vi "M81 Read Values_Suslov.vi"(9 "Slot":enum32{"Slot 1", "Slot 2", "Slot 3"}(ring), 10 "Command string":string, 11 "VISA resource name":refnum<visa-resource-name>) -> (2 "Resistance":dbl[](array[numeric]), 3 "VISA resource name":refnum<visa-resource-name>)   [LabVIEW 2025]
doc: "Author: Scott Hannahs <sth@magnet.fsu.edu>\n\nThis software is licensed for use under the “MIT License\"\nCopyright (c) 2025 Scott Hannahs, sth@sth@magnet.sthnet.net\n\nPermission is hereby granted, free of charge, to any person obtaining a copy of this software and associated documentation files (the \"Software\"), to deal in the Software without restriction, including without limitation the rights to use, copy, modify, merge, publish, distribute, sublicense, and/or sell copies of the Software, and to permit persons to whom the Software is furnished to do so, subject to the following conditions: The above copyright notice and this permission notice shall be included in all copies or substantial portions of the Software.\n\nTHE SOFTWARE IS PROVIDED \"AS IS\", WITHOUT WARRANTY OF ANY KIND, EXPRESS OR IMPLIED, INCLUDING BUT NOT LIMITED TO THE WARRANTIES OF MERCHANTABILITY, FITNESS FOR A PARTICULAR PURPOSE AND NONINFRINGEMENT. IN NO EVENT SHALL THE AUTHORS OR COPYRIGHT HOLDERS BE LIABLE FOR ANY CLAIM, DAMAGES OR OTHER LIABILITY, WHETHER IN AN ACTION OF CONTRACT, TORT OR OTHERWISE, ARISING FROM, OUT OF OR IN CONNECTION WITH THE SOFTWARE OR THE USE OR OTHER DEALINGS IN THE SOFTWARE."
panel:
  in  "Wait (ms)":u32=30
  out "String Response":string
  out "Error Out":errorcluster
  in  "Error In":errorcluster
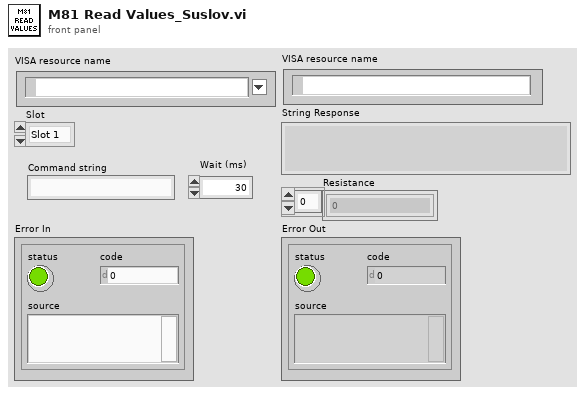
[diagram p1: front panel]
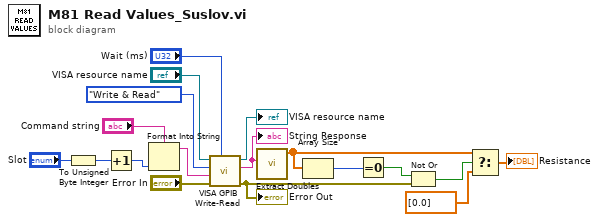
[diagram p0: block diagram]
diagram:
  n1 = To Unsigned Byte Integer(number="Slot") -> (unsigned 8bit integer=w1:u8)
  n2 = Increment(x=w1) -> (x+1=w4:u8)
  n3 = Format Into String(format string="Command string", w4) -> (resulting string=w2:string)  [unwired: 2 in, 1 out]
  n4 = call "VISA GPIB Write-Read.vi"("Wait (ms)"="Wait (ms)", "error in (no error)"="Error In", "Command"=w2, "Action"=enum16{"Write", "Read", "Write & Read"}."Write & Read", "VISA resource name"="VISA resource name") -> ("error out"=w10:errorcluster, "String Returned"=w5:string, "dup VISA Session"=→"VISA resource name":refnum<visa-resource-name>)  [unwired: 3 in, 1 out]
  "Error Out" <- w10
  "String Response" <- w5
  n5 = call "Extract Doubles.vi"("String"=w5) -> ("Data"=w16:dbl[])  [unwired: 5 in, 1 out]
  n6 = Array Size(array=w16) -> (size(s)=w13:i32)
  n7 = Equal To 0?(x=w13) -> (x = 0?=w14:bool)
  n8 = Not Or(1:w10, 2:w14) -> (0:w15:bool)
  n9 = Select(t=w16, s=w15, f=dbl[] [0.0]) -> (s? t:f=→"Resistance":dbl[])
